vi "XY图数据提取.vi"(4 "XY对":T1, 5 "输入数据":T2(array[cluster])) -> (1 "提取后XY对数组":cluster{dbl, dbl}[](array[cluster]))   [LabVIEW 2018]
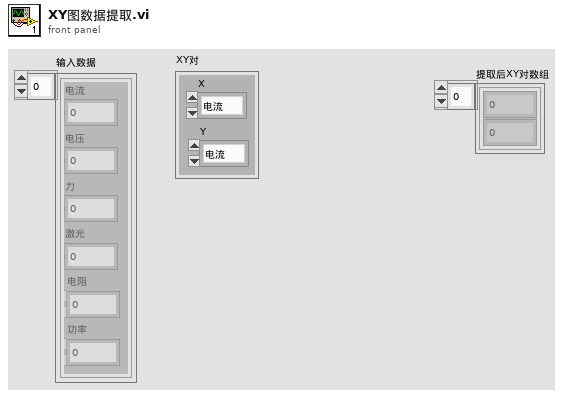
[diagram p1: front panel]
types:
  T1 = cluster{"X":enum16{"电流", "电压", "力", "位移", "电阻", "功率", "测试"}, "Y":enum16{"电流", "电压", "力", "位移", "电阻", "功率", "测试"}}
  T2 = cluster{"电流":dbl, "电压":dbl, "力":dbl, "激光":dbl, "电阻":dbl, "功率":dbl}[]
  T3 = cluster{"电流":dbl, "电压":dbl, "力":dbl, "激光":dbl, "电阻":dbl, "功率":dbl}
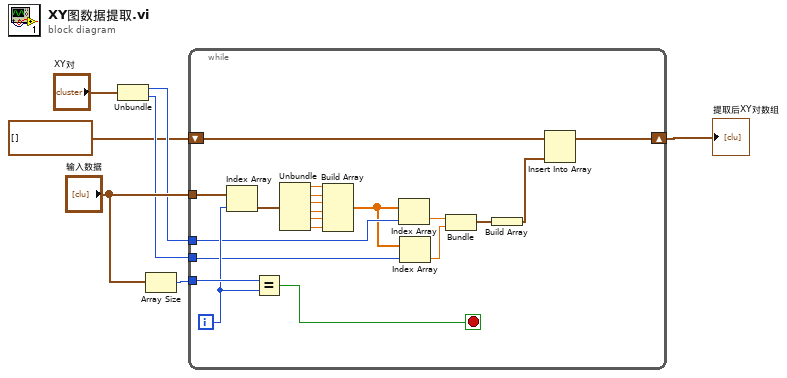
[diagram p0: block diagram]
diagram:
  n1 = Unbundle("XY对") -> ("X"=w4:enum16{"电流", "电压", "力", "位移", "电阻", "功率", "测试"}, "Y"=w3:enum16{"电流", "电压", "力", "位移", "电阻", "功率", "测试"})
  n2 = Array Size(array="输入数据") -> (size(s)=w7:i32)
  n3 = while {
    tunnel: w7 -> [w27]
    tunnel: "输入数据" -> [w25]
    tunnel: w4 -> [w16]
    tunnel: w3 -> [w14]
    shift-right: [w8] -> w1
    shift-left: cluster{dbl, dbl}[] [] -> [w10]
    i -> [w24]
    stop <- w26 stop-if-true
    n4 = Index Array(array=w25, index=w24) -> (element=w23:T3)
    n5 = Equal?(x=w27, y=w24) -> (x = y?=w26:bool)
    n6 = Unbundle(w23) -> ("电流"=w22:dbl, "电压"=w17:dbl, "力"=w18:dbl, "激光"=w19:dbl, "电阻"=w20:dbl, "功率"=w21:dbl)
    n7 = Build Array(w22, w17, w18, w19, w20, w21) -> (w15:dbl[])
    n8 = Index Array(array=w15, index=w16) -> (element=w13:dbl)
    n9 = Index Array(array=w15, index=w14) -> (element=w12:dbl)
    n10 = Bundle("功率"=w13, "功率"=w12) -> (w11:cluster{"功率":dbl, "功率":dbl})  [unwired: 1 in]
    n11 = Build Array(w11) -> (w9:cluster{"功率":dbl, "功率":dbl}[])
    n12 = Insert Into Array(array=w10, new element=w9) -> (w8:cluster{dbl, dbl}[])  [unwired: 1 in]
  }
  "提取后XY对数组" <- w1
